vi "Write Ctl Refnum.vi"(8 "error in (no error)":errorcluster, 10 "Ctl Refnum":refnum<vi>, 11 "String Control in":refnum<class "String Control.lvclass">) -> (0 "error out":errorcluster, 3 "String Control out":refnum<class "String Control.lvclass">)   [LabVIEW 2010, in "String Control.lvclass"]
uses:
  String Control.lvclass
  String Control.lvclass/String Control.ctl
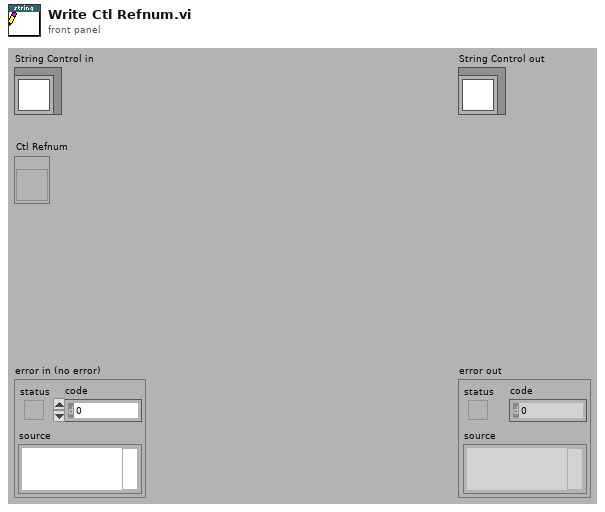
[diagram p1: front panel]
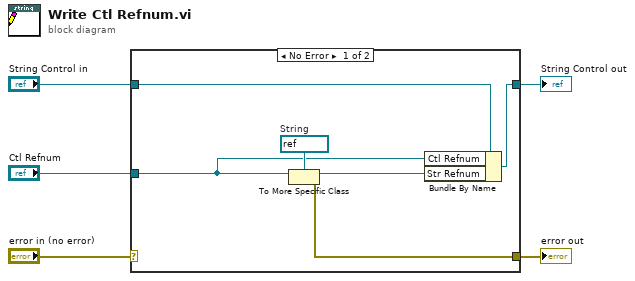
[diagram p0: block diagram]
diagram:
  n1 = case shown="No Error" "error in (no error)" {
    selector: "error in (no error)" -> [_ w12]
    tunnel: [w7 w12] -> w4
    tunnel: [w10 w13] -> w2
    tunnel: "String Control in" -> [w11 w13]
    tunnel: "Ctl Refnum" -> [w6 _]
    frame No Error {
      w9 = refnum<vi> refnum  # String
      n2 = To More Specific Class(target class=w9, reference=w6) -> (specific class reference=w8:refnum<vi>, error out=w7:errorcluster)  [unwired: 1 in]
      n3 = Bundle By Name(cluster=w11, "Ctl Refnum"=w6, "Str Refnum"=w8) -> (w10:refnum<class "String Control.lvclass">)
    }
    frame Error {
    }
  }
  "error out" <- w4
  "String Control out" <- w2
